vi "数组时间戳格式化(子VI).vi"(11 "待发送数据输入":string[][](array[string])) -> (3 "待发送数据输出":string[][](array[string]))   [LabVIEW 2016, in "数据传输系统.lvlib"]
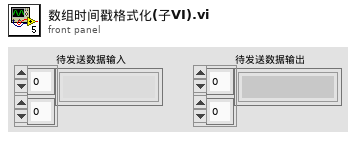
[diagram p1: front panel]
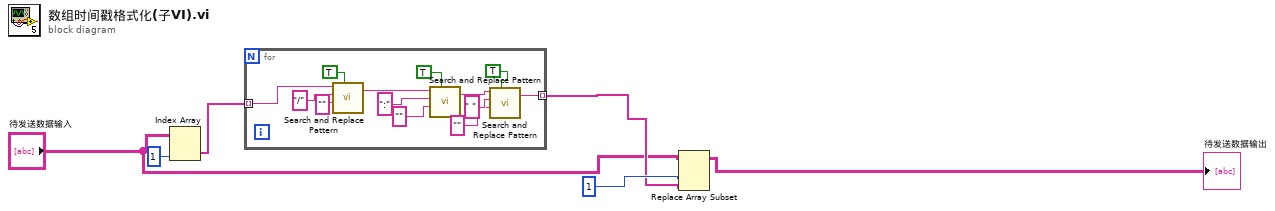
[diagram p0: block diagram]
diagram:
  n1 = Index Array(array="待发送数据输入", index (col)=1 ("禁用的索引 (列)")) -> (element=w2:string[])  [unwired: 1 in]
  n2 = for {
    tunnel: w2 -> [w19] mode=indexing
    tunnel: [w11] -> w4 mode=indexing
    n3 = call <vilib>:"Search and Replace Pattern.vi"("string"=w19, "regular expression (\"\")"="/" ("子字符串(\"\")"), "replace string (\"\")"="" ("replace string (\"\")"), "replace all? (F)"=TRUE ("替换全部？(F)")) -> ("result string"=w15:string)  [unwired: 1 in, 1 out]
    n4 = call <vilib>:"Search and Replace Pattern.vi"("string"=w15, "regular expression (\"\")"=":" ("子字符串(\"\")"), "replace string (\"\")"="" ("replace string (\"\")"), "replace all? (F)"=TRUE ("替换全部？(F)")) -> ("result string"=w10:string)  [unwired: 1 in, 1 out]
    n5 = call <vilib>:"Search and Replace Pattern.vi"("string"=w10, "regular expression (\"\")"=" " ("子字符串(\"\")"), "replace string (\"\")"="" ("replace string (\"\")"), "replace all? (F)"=TRUE ("替换全部？(F)")) -> ("result string"=w11:string)  [unwired: 1 in, 1 out]
  }
  n6 = Replace Array Subset(array="待发送数据输入", new element=w4, index (col)=1 ("禁用的索引 (列)")) -> (→"待发送数据输出":string[][])  [unwired: 1 in]
